vi "Add Structure to Cache.vi"(8 "error in":errorcluster, 9 "SREF":string, 10 "Geometric In":refnum<class "Geometric.lvclass">[](array[class]), 11 "ParseGDSII in":refnum<class "ParseGDSII.lvclass">) -> (0 "error out":errorcluster, 2 "Geometric Out":refnum<class "Geometric.lvclass">[](array[class]), 3 "ParseGDSII out":refnum<class "ParseGDSII.lvclass">)   [LabVIEW 2019, in "ParseGDSII.lvclass"]
uses:
  ParseGDSII.lvclass
  Elements/Geometric.lvclass
  Structures/Structure.lvclass
  ParseGDSII.lvclass/ParseGDSII.ctl
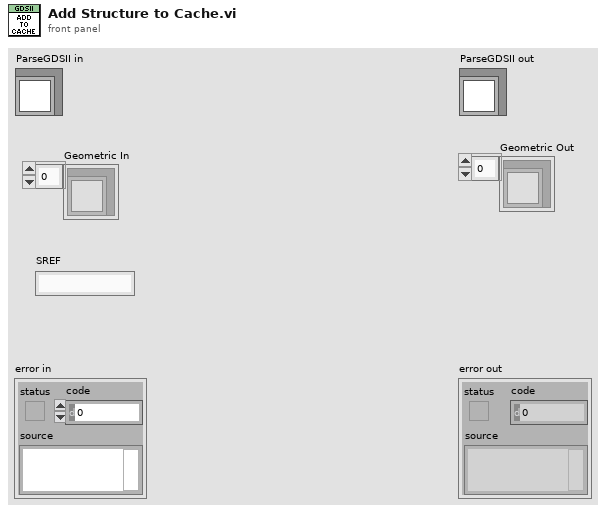
[diagram p1: front panel]
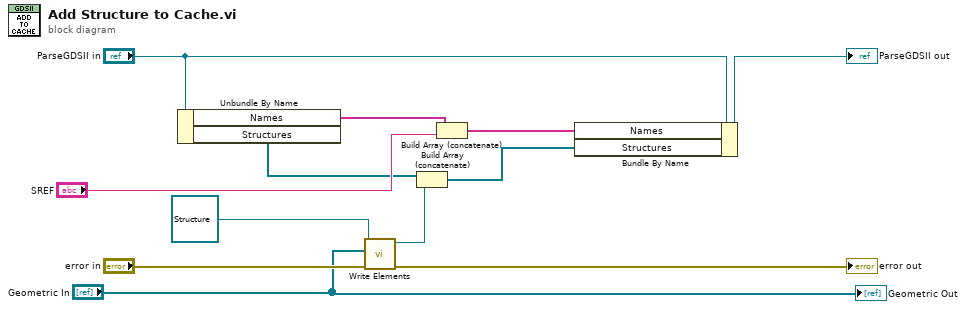
[diagram p0: block diagram]
diagram:
  n1 = Unbundle By Name("ParseGDSII in") -> ("Names"=w10:string[], "Structures"=w5:refnum<class "Structure.lvclass">[])
  n2 = call "Write Elements.vi"("error in (no error)"="error in", "Elements"="Geometric In", "Structure.lvclass in"=refnum<class "Structure.lvclass"> refnum) -> ("error out"=→"error out":errorcluster, "Structure.lvclass out"=w7:refnum<class "Structure.lvclass">)  [unwired: 7 in]
  n3 = Build Array (concatenate)(w5, w7) -> (w6:refnum<class "Structure.lvclass">[])
  n4 = Build Array (concatenate)(w10, "SREF") -> (w9:string[])
  n5 = Bundle By Name(cluster="ParseGDSII in", "Names"=w9, "Structures"=w6) -> (→"ParseGDSII out":refnum<class "ParseGDSII.lvclass">)
  "Geometric Out" <- "Geometric In"
